vi "Get Server State Ref.vi"(11 "Template Server in":refnum<class "Ex1_server.lvclass">) -> (2 "Server State Ref":refnum<data-value>, 3 "Template Server out":refnum<class "Ex1_server.lvclass">)   [LabVIEW 2019, in "Ex1_server.lvlib" / "Ex1_server.lvclass"]
uses:
  Ex1_server.lvclass
  typeDefs/Server State Data.ctl
  Ex1_server.lvclass/Ex1_server.ctl
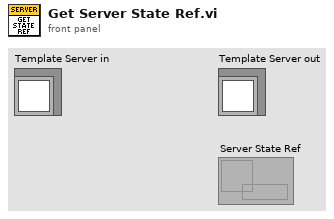
[diagram p1: front panel]
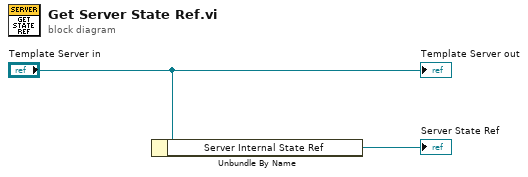
[diagram p0: block diagram]
diagram:
  n1 = Unbundle By Name("Template Server in") -> ("Server Internal State Ref"=→"Server State Ref":refnum<data-value>)
  "Template Server out" <- "Template Server in"
